vi "GlueDispenseTester.vi"() -> ()   [LabVIEW 2021]
panel:
  out "Time(ms)":dbl
  out "Speed":dbl format="%#_13g"
  out "Comm":string
  in  "Z":dbl=71.609 format="%#_13g"
  in  "Pressure":dbl[](array[numeric])=[27.0, 27.0, 27.0, 27.0]
  in  "Path":path=path "C:/Users/TTUHEP/Documents/LabVIEW/GantryPrograms/include/DispenserTools/SH_V3_try13_CirclesANDLinesANDEdge_3LAYERS_F48_ROTATED_11-22-2022_EdgesModified_InnerLinesModified_CirclesModified_notchesfixed_Z7mm_Stage1.ngc"
  in  "Serial Configuration":T1={"Baud Rate "=115200, "Parity "=0, "Data Bits "=8, "Stop Bits"=10} {"Stop Bits" items=["1.0"=10, "1.5"=15, "2.0"=20]; "Data Bits" items=["7"=7, "8"=8]; "Parity" items=["None", "Odd", "Even"]; "Baud Rate" items=["9600"=9600, "19200"=19200, "38400"=38400, "115200"=115200]}
  in  "Y":dbl=905.746 format="%#_13g"
  in  "X":dbl=435.404 format="%#_13g"
  in  "VISA resource name":refnum<visa-resource-name>="COM6"
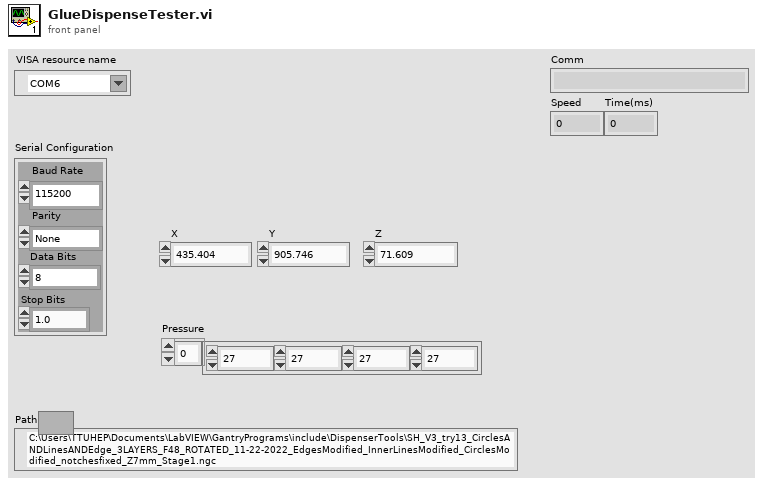
[diagram p1: front panel]
types:
  T1 = cluster{"Baud Rate ":u32, "Parity ":u16, "Data Bits ":u16, "Stop Bits":u16}
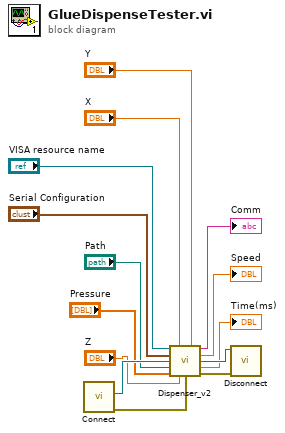
[diagram p0: block diagram]
diagram:
  n1 = call "Connect.vi"() -> ("error out"=w13:errorcluster, "controller"=w14:refnum<k24>)  [unwired: 10 in]
  n2 = call "Dispenser_v2.vi"("VISA resource name"="VISA resource name", "X"="X", "Y"="Y", "Serial Configuration"="Serial Configuration", "controller in"=w14, "Path"="Path", "Pressure"="Pressure", "Z"="Z", "error in (no error)"=w13) -> ("Comm"=→"Comm":string, "Speed"=→"Speed":dbl, "controller out"=w11:refnum<k24>, "Time(ms)"=→"Time(ms)":dbl, "error out"=w12:errorcluster)  [unwired: 2 in]
  n3 = call "Disconnect.vi"("error in (no error)"=w12, "controller"=w11) -> ()  [unwired: 9 in, 1 out]
